vi "Untitled 1 (SubVI).vi"(10 "dt (ms)":u32, 11 "Numeric":i32) -> ()   [LabVIEW 2016]
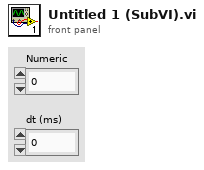
[diagram p1: front panel]
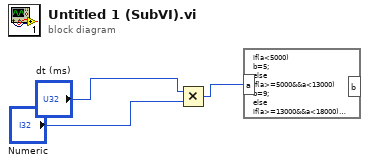
[diagram p0: block diagram]
diagram:
  n1 = Multiply(x="dt (ms)", y="Numeric") -> (x*y=w3:u32)
  n2 = formula code="if(a<5000)\nb=5;\nelse \nif(a>=5000&&a<13000)\nb=9;\nelse\nif(a>=13000&&a<18000)\nb=13;\nelse\nif(a>=18000&&a<23000)\nb=7;\nelse\nif(a>=23000&&a<23000)\nb=-8;\nelse\nif(a>=23000)\nb=0;"("a"=w3) -> ()  [unwired: 1 out]
